vi "solar_voy_def Import (Item_Def).vi"(10 "Arguments":string[](array[string]), 11 "Item Tag":string) -> (1 "Valid?":bool, 2 "ID":u16, 3 "ITEM":T1)   [LabVIEW 2018]
doc: "This imports COSMOS parameter/item tag. Refer to: http://cosmosrb.com/docs/cmdtlm/\n\nSupported tags: \nPARAMETER\nARRAY_PARAMETER\nITEM, ARRAY_ITEM\nID_PARAMETER\nID_ITEM\nAPPEND_PARAMETER\nAPPEND_ARRAY_PARAMETER\nAPPEND_ARRAY_ITEM\nAPPEND_ID_PARAMETER\nAPPEND_ID_ITEM"
uses:
  type/solar_type Item Type.ctl
  solar_voy_def_ctl ITEM TYPE.ctl
  solar_voy_def_ctl ITEM.ctl
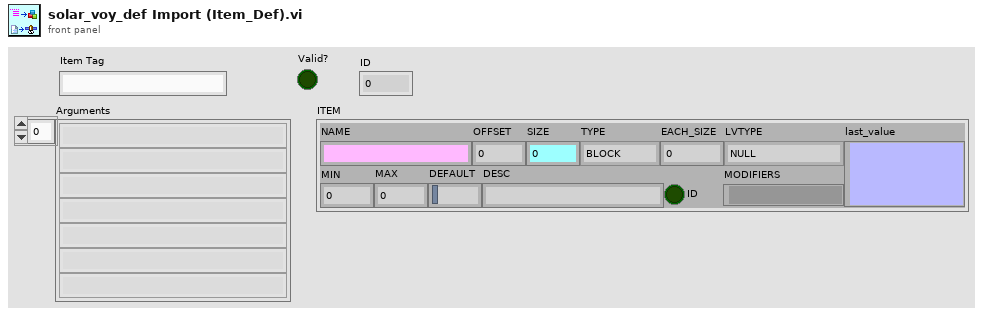
[diagram p1: front panel]
types:
  T1 = typedef "solar_voy_def_ctl ITEM.ctl" = cluster{"NAME":string, "OFFSET":i32, "SIZE":i32, "TYPE":T2, "EACH_SIZE":i32, "LVTYPE":T3, "MIN":dbl, "MAX":dbl, "DEFAULT":string, "DESC":string, "ID":bool, "MODIFIERS":variant, "last_value":variant}
  T2 = typedef "solar_voy_def_ctl ITEM TYPE.ctl" = enum8{"BLOCK", "INT", "UINT", "FLOAT", "STRING"}
  T3 = typedef "solar_type Item Type.ctl" = enum16{"NULL", "UNKNOWN", "CLUSTER", "I8", "I16", "I32", "I64", "U8", "U16", "U32", "U64", "U8_ENUM", "U16_ENUM", "U32_ENUM", "SGL", "DBL", "BOOLEAN", "STRING", "PATH", "VISA", "TAG", "TIME", "I8_1D", "I16_1D", "I32_1D", "I64_1D", "U8_1D", "U16_1D", "U32_1D", "U64_1D", "U8_ENUM_1D", "U16_ENUM_1D", "U32_ENUM_1D", "SGL_1D", "DBL_1D", "BOOLEAN_1D", "STRING_1D", "PATH_1D", "VISA_1D", "TAG_1D", "TIME_1D", "I8_2D", "I16_2D", "I32_2D", "I64_2D", "U8_2D", "U16_2D", "U32_2D", "U64_2D", "U8_ENUM_2D", "U16_ENUM_2D", "U32_ENUM_2D", "SGL_2D", "DBL_2D", "BOOLEAN_2D", "STRING_2D", "PATH_2D", "VISA_2D", "TAG_2D", "TIME_2D"}
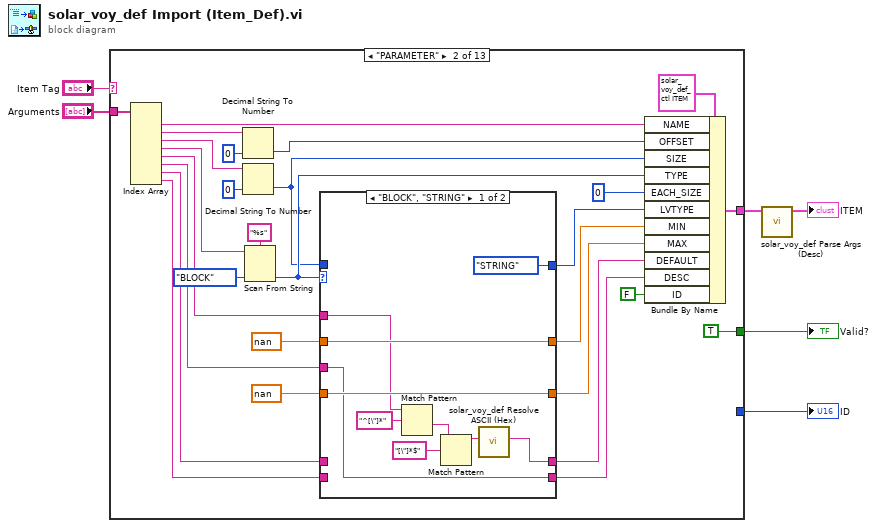
[diagram p0: block diagram]
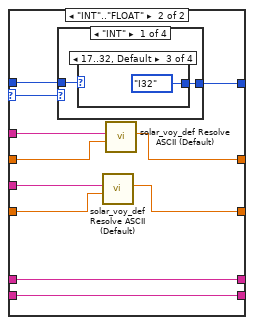
[diagram p3: hidden frame]
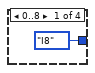
[diagram p4: hidden frame]
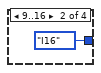
[diagram p5: hidden frame]
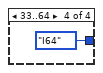
[diagram p6: hidden frame]
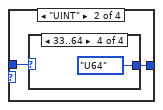
[diagram p7: hidden frame]
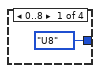
[diagram p8: hidden frame]
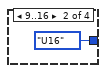
[diagram p9: hidden frame]
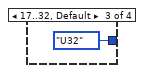
[diagram p10: hidden frame]
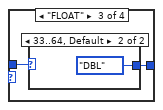
[diagram p11: hidden frame]
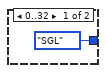
[diagram p12: hidden frame]
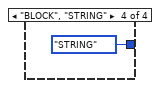
[diagram p13: hidden frame]
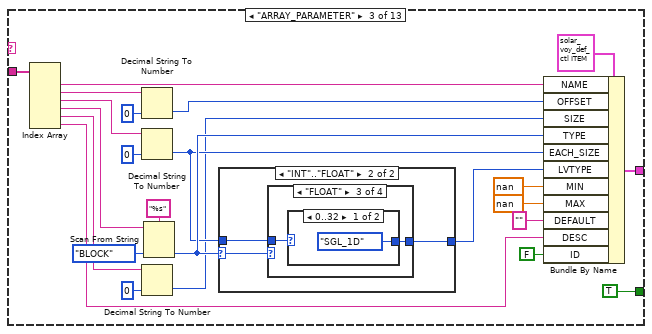
[diagram p14: hidden frame]
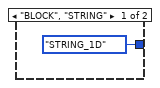
[diagram p15: hidden frame]
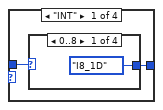
[diagram p16: hidden frame]
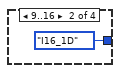
[diagram p17: hidden frame]
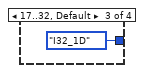
[diagram p18: hidden frame]
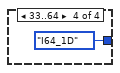
[diagram p19: hidden frame]
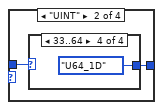
[diagram p20: hidden frame]
diagram:
  n1 = case shown="\"PARAMETER\"" "Item Tag" {
    tunnel: "Arguments" -> [_ w25 w93 w136 w181 w227 w299 w352 w418 w461 w502 w546 w616]
    tunnel: [_ w10 w84 w125 w172 w213 w288 w340 w412 w455 w494 w534 w608] -> w1
    tunnel: [_ TRUE TRUE TRUE TRUE TRUE TRUE TRUE TRUE TRUE TRUE TRUE TRUE] -> w4
    tunnel: [_ _ _ _ _ w206 w280 _ _ _ _ w526 w599] -> w3
    frame Default {
    }
    frame "PARAMETER" {
      n2 = Index Array(array=w25) -> (element #1=w24:string, element #2=w26:string, element #3=w27:string, element #4=w28:string, element #5=w29:string, element #6=w30:string, element #7=w32:string, element #8=w34:string)  [unwired: 8 in]
      n3 = Decimal String To Number(string=w26, default (0L)=0 ("OFFSET")) -> (number=w13:i32)  [unwired: 1 in, 1 out]
      n4 = Decimal String To Number(string=w27, default (0L)=0 ("OFFSET")) -> (number=w17:i32)  [unwired: 1 in, 1 out]
      n5 = Scan From String(format string="%s", input string=w28, default 1=solar_voy_def_ctl_ITEM_TYPE."BLOCK" ("TYPE")) -> (output 1=w22:T2)  [unwired: 2 in, 3 out]
      n6 = case shown="\"BLOCK\", \"STRING\"" w22 {
        selector: w22 -> [_ w53]
        tunnel: w17 -> [_ w55]
        tunnel: [solar_type_Item_Type."STRING" ("LVTYPE") w54] -> w18
        tunnel: nan ("MIN") -> [w43 w49]
        tunnel: [w43 w48] -> w20
        tunnel: nan ("MIN") -> [w42 w46]
        tunnel: [w42 w45] -> w23
        tunnel: w29 -> [w40 w50]
        tunnel: w30 -> [w41 w47]
        tunnel: [w35 w52] -> w31
        tunnel: w32 -> [_ w52]
        tunnel: [w41 w51] -> w33
        tunnel: w34 -> [_ w51]
        frame "BLOCK", "STRING" {
          n7 = Match Pattern(string=w40, regular expression="^[\"]*") -> (after substring=w38:string)  [unwired: 1 in, 3 out]
          n8 = Match Pattern(string=w38, regular expression="[\"]*$") -> (before substring=w36:string)  [unwired: 1 in, 3 out]
          n9 = call "solar_voy_def Resolve ASCII (Hex).vi"("DEFAULT (ASCII '\\xFF')"=w36) -> ("Resolved DEFAULT (Hex 'xFF')"=w35:string)  [unwired: 10 in]
        }
        frame "INT".."FLOAT" {
          n10 = case shown="\"INT\"" w53 {
            tunnel: w55 -> [w57 w63 w69 _]
            tunnel: [w56 w62 w68 solar_type_Item_Type."STRING" ("LVTYPE")] -> w54
            frame "INT" {
              n11 = case shown="17..32, Default" w57 {
                tunnel: [solar_type_Item_Type."I8" ("LVTYPE") solar_type_Item_Type."I16" ("LVTYPE") solar_type_Item_Type."I32" ("LVTYPE") solar_type_Item_Type."I64" ("LVTYPE")] -> w56
                frame 0..8 {
                }
                frame 9..16 {
                }
                frame 17..32, Default {
                }
                frame 33..64 {
                }
              }
            }
            frame "UINT" {
              n12 = case shown="33..64" w63 {
                tunnel: [solar_type_Item_Type."U8" ("LVTYPE") solar_type_Item_Type."U16" ("LVTYPE") solar_type_Item_Type."U32" ("LVTYPE") solar_type_Item_Type."U64" ("LVTYPE")] -> w62
                frame 0..8 {
                }
                frame 9..16 {
                }
                frame 17..32, Default {
                }
                frame 33..64 {
                }
              }
            }
            frame "FLOAT" {
              n13 = case shown="33..64, Default" w69 {
                tunnel: [solar_type_Item_Type."SGL" ("LVTYPE") solar_type_Item_Type."DBL" ("LVTYPE")] -> w68
                frame 0..32 {
                }
                frame 33..64, Default {
                }
              }
            }
            frame "BLOCK", "STRING" {
            }
          }
          n14 = call "solar_voy_def Resolve ASCII (Default).vi"("Default (NaN=Use Default)"=w46, "DEFAULT,MIN,MAX"=w47) -> ("DEFAULT,MIN,MAX out"=w45:dbl)  [unwired: 9 in]
          n15 = call "solar_voy_def Resolve ASCII (Default).vi"("Default (NaN=Use Default)"=w49, "DEFAULT,MIN,MAX"=w50) -> ("DEFAULT,MIN,MAX out"=w48:dbl)  [unwired: 9 in]
        }
      }
      n16 = Bundle By Name(cluster=T1 {"NAME"="", "OFFSET"=0, "SIZE"=0, "TYPE"=enum."BLOCK", "EACH_SIZE"=0, "LVTYPE"=enum."NULL", "MIN"=0.0, "MAX"=0.0, "DEFAULT"="", "DESC"="", "ID"=FALSE, "MODIFIERS"=variant, "last_value"=variant} ("element"), "NAME"=w24, "OFFSET"=w13, "SIZE"=w17, "TYPE"=w22, "EACH_SIZE"=0, "LVTYPE"=w18, "MIN"=w20, "MAX"=w23, "DEFAULT"=w31, "DESC"=w33, "ID"=FALSE) -> (w10:T1)
    }
    frame "ARRAY_PARAMETER" {
      n17 = Index Array(array=w93) -> (element #1=w92:string, element #2=w94:string, element #3=w95:string, element #4=w96:string, element #5=w78:string, element #6=w76:string)  [unwired: 6 in]
      n18 = Decimal String To Number(string=w94, default (0L)=0 ("OFFSET")) -> (number=w86:i32)  [unwired: 1 in, 1 out]
      n19 = Decimal String To Number(string=w95, default (0L)=0 ("OFFSET")) -> (number=w80:i32)  [unwired: 1 in, 1 out]
      n20 = Decimal String To Number(string=w78, default (0L)=0 ("OFFSET")) -> (number=w77:i32)  [unwired: 1 in, 1 out]
      n21 = Scan From String(format string="%s", input string=w96, default 1=solar_voy_def_ctl_ITEM_TYPE."BLOCK" ("TYPE")) -> (output 1=w91:T2)  [unwired: 2 in, 3 out]
      n22 = case shown="\"INT\"..\"FLOAT\"" w91 {
        selector: w91 -> [_ w98]
        tunnel: w80 -> [_ w100]
        tunnel: [solar_type_Item_Type."STRING_1D" ("LVTYPE") w99] -> w90
        frame "BLOCK", "STRING" {
        }
        frame "INT".."FLOAT" {
          n23 = case shown="\"FLOAT\"" w98 {
            tunnel: w100 -> [w102 w108 w114 _]
            tunnel: [w101 w107 w113 solar_type_Item_Type."STRING" ("LVTYPE")] -> w99
            frame "INT" {
              n24 = case shown="0..8" w102 {
                tunnel: [solar_type_Item_Type."I8_1D" ("LVTYPE") solar_type_Item_Type."I16_1D" ("LVTYPE") solar_type_Item_Type."I32_1D" ("LVTYPE") solar_type_Item_Type."I64_1D" ("LVTYPE")] -> w101
                frame 0..8 {
                }
                frame 9..16 {
                }
                frame 17..32, Default {
                }
                frame 33..64 {
                }
              }
            }
            frame "UINT" {
              n25 = case shown="33..64" w108 {
                tunnel: [solar_type_Item_Type."U8_1D" ("LVTYPE") solar_type_Item_Type."U16_1D" ("LVTYPE") solar_type_Item_Type."U32_1D" ("LVTYPE") solar_type_Item_Type."U64_1D" ("LVTYPE")] -> w107
                frame 0..8 {
                }
                frame 9..16 {
                }
                frame 17..32, Default {
                }
                frame 33..64 {
                }
              }
            }
            frame "FLOAT" {
              n26 = case shown="0..32" w114 {
                tunnel: [solar_type_Item_Type."SGL_1D" ("LVTYPE") solar_type_Item_Type."DBL_1D" ("LVTYPE")] -> w113
                frame 0..32 {
                }
                frame 33..64, Default {
                }
              }
            }
            frame "BLOCK", "STRING" {
            }
          }
        }
      }
      n27 = Bundle By Name(cluster=T1 {"NAME"="", "OFFSET"=0, "SIZE"=0, "TYPE"=enum."BLOCK", "EACH_SIZE"=0, "LVTYPE"=enum."NULL", "MIN"=0.0, "MAX"=0.0, "DEFAULT"="", "DESC"="", "ID"=FALSE, "MODIFIERS"=variant, "last_value"=variant} ("element"), "NAME"=w92, "OFFSET"=w86, "SIZE"=w77, "TYPE"=w91, "EACH_SIZE"=w80, "LVTYPE"=w90, "MIN"=nan, "MAX"=nan ("MIN"), "DEFAULT"="", "DESC"=w76, "ID"=FALSE) -> (w84:T1)
    }
    frame "ITEM" {
      n28 = Index Array(array=w136) -> (element #1=w135:string, element #2=w137:string, element #3=w138:string, element #4=w139:string, element #5=w118:string)  [unwired: 5 in]
      n29 = Decimal String To Number(string=w137, default (0L)=0 ("OFFSET")) -> (number=w128:i32)  [unwired: 1 in, 1 out]
      n30 = Decimal String To Number(string=w138, default (0L)=0 ("OFFSET")) -> (number=w132:i32)  [unwired: 1 in, 1 out]
      n31 = Scan From String(format string="%s", input string=w139, default 1=solar_voy_def_ctl_ITEM_TYPE."BLOCK" ("TYPE")) -> (output 1=w134:T2)  [unwired: 2 in, 3 out]
      n32 = case shown="\"INT\"..\"FLOAT\"" w134 {
        selector: w134 -> [_ w141]
        tunnel: w132 -> [_ w143]
        tunnel: [solar_type_Item_Type."STRING" ("LVTYPE") w142] -> w133
        frame "BLOCK", "STRING" {
        }
        frame "INT".."FLOAT" {
          n33 = case shown="\"INT\"" w141 {
            tunnel: w143 -> [w145 w151 w157 _]
            tunnel: [w144 w150 w156 solar_type_Item_Type."STRING" ("LVTYPE")] -> w142
            frame "INT" {
              n34 = case shown="17..32, Default" w145 {
                tunnel: [solar_type_Item_Type."I8" ("LVTYPE") solar_type_Item_Type."I16" ("LVTYPE") solar_type_Item_Type."I32" ("LVTYPE") solar_type_Item_Type."I64" ("LVTYPE")] -> w144
                frame 0..8 {
                }
                frame 9..16 {
                }
                frame 17..32, Default {
                }
                frame 33..64 {
                }
              }
            }
            frame "UINT" {
              n35 = case shown="33..64" w151 {
                tunnel: [solar_type_Item_Type."U8" ("LVTYPE") solar_type_Item_Type."U16" ("LVTYPE") solar_type_Item_Type."U32" ("LVTYPE") solar_type_Item_Type."U64" ("LVTYPE")] -> w150
                frame 0..8 {
                }
                frame 9..16 {
                }
                frame 17..32, Default {
                }
                frame 33..64 {
                }
              }
            }
            frame "FLOAT" {
              n36 = case shown="33..64, Default" w157 {
                tunnel: [solar_type_Item_Type."SGL" ("LVTYPE") solar_type_Item_Type."DBL" ("LVTYPE")] -> w156
                frame 0..32 {
                }
                frame 33..64, Default {
                }
              }
            }
            frame "BLOCK", "STRING" {
            }
          }
        }
      }
      n37 = Bundle By Name(cluster=T1 {"NAME"="", "OFFSET"=0, "SIZE"=0, "TYPE"=enum."BLOCK", "EACH_SIZE"=0, "LVTYPE"=enum."NULL", "MIN"=0.0, "MAX"=0.0, "DEFAULT"="", "DESC"="", "ID"=FALSE, "MODIFIERS"=variant, "last_value"=variant} ("element"), "NAME"=w135, "OFFSET"=w128, "SIZE"=w132, "TYPE"=w134, "EACH_SIZE"=0, "LVTYPE"=w133, "MIN"=nan, "MAX"=nan ("MIN"), "DEFAULT"="", "DESC"=w118, "ID"=FALSE) -> (w125:T1)
    }
    frame "ARRAY_ITEM" {
      n38 = Index Array(array=w181) -> (element #1=w180:string, element #2=w182:string, element #3=w183:string, element #4=w184:string, element #5=w166:string, element #6=w164:string)  [unwired: 6 in]
      n39 = Decimal String To Number(string=w182, default (0L)=0 ("OFFSET")) -> (number=w174:i32)  [unwired: 1 in, 1 out]
      n40 = Decimal String To Number(string=w183, default (0L)=0 ("OFFSET")) -> (number=w168:i32)  [unwired: 1 in, 1 out]
      n41 = Decimal String To Number(string=w166, default (0L)=0 ("OFFSET")) -> (number=w165:i32)  [unwired: 1 in, 1 out]
      n42 = Scan From String(format string="%s", input string=w184, default 1=solar_voy_def_ctl_ITEM_TYPE."BLOCK" ("TYPE")) -> (output 1=w179:T2)  [unwired: 2 in, 3 out]
      n43 = case shown="\"INT\"..\"FLOAT\"" w179 {
        selector: w179 -> [_ w186]
        tunnel: w168 -> [_ w188]
        tunnel: [solar_type_Item_Type."STRING_1D" ("LVTYPE") w187] -> w178
        frame "BLOCK", "STRING" {
        }
        frame "INT".."FLOAT" {
          n44 = case shown="\"FLOAT\"" w186 {
            tunnel: w188 -> [w190 w196 w202 _]
            tunnel: [w189 w195 w201 solar_type_Item_Type."STRING" ("LVTYPE")] -> w187
            frame "INT" {
              n45 = case shown="0..8" w190 {
                tunnel: [solar_type_Item_Type."I8_1D" ("LVTYPE") solar_type_Item_Type."I16_1D" ("LVTYPE") solar_type_Item_Type."I32_1D" ("LVTYPE") solar_type_Item_Type."I64_1D" ("LVTYPE")] -> w189
                frame 0..8 {
                }
                frame 9..16 {
                }
                frame 17..32, Default {
                }
                frame 33..64 {
                }
              }
            }
            frame "UINT" {
              n46 = case shown="33..64" w196 {
                tunnel: [solar_type_Item_Type."U8_1D" ("LVTYPE") solar_type_Item_Type."U16_1D" ("LVTYPE") solar_type_Item_Type."U32_1D" ("LVTYPE") solar_type_Item_Type."U64_1D" ("LVTYPE")] -> w195
                frame 0..8 {
                }
                frame 9..16 {
                }
                frame 17..32, Default {
                }
                frame 33..64 {
                }
              }
            }
            frame "FLOAT" {
              n47 = case shown="0..32" w202 {
                tunnel: [solar_type_Item_Type."SGL_1D" ("LVTYPE") solar_type_Item_Type."DBL_1D" ("LVTYPE")] -> w201
                frame 0..32 {
                }
                frame 33..64, Default {
                }
              }
            }
            frame "BLOCK", "STRING" {
            }
          }
        }
      }
      n48 = Bundle By Name(cluster=T1 {"NAME"="", "OFFSET"=0, "SIZE"=0, "TYPE"=enum."BLOCK", "EACH_SIZE"=0, "LVTYPE"=enum."NULL", "MIN"=0.0, "MAX"=0.0, "DEFAULT"="", "DESC"="", "ID"=FALSE, "MODIFIERS"=variant, "last_value"=variant} ("element"), "NAME"=w180, "OFFSET"=w174, "SIZE"=w165, "TYPE"=w179, "EACH_SIZE"=w168, "LVTYPE"=w178, "MIN"=nan, "MAX"=nan ("MIN"), "DEFAULT"="", "DESC"=w164, "ID"=FALSE) -> (w172:T1)
    }
    frame "ID_PARAMETER" {
      n49 = Index Array(array=w227) -> (element #1=w226:string, element #2=w228:string, element #3=w229:string, element #4=w230:string, element #5=w231:string, element #6=w232:string, element #7=w233:string, element #8=w235:string)  [unwired: 8 in]
      n50 = Decimal String To Number(string=w228, default (0L)=0 ("OFFSET")) -> (number=w216:i32)  [unwired: 1 in, 1 out]
      n51 = Decimal String To Number(string=w229, default (0L)=0 ("OFFSET")) -> (number=w209:i32)  [unwired: 1 in, 1 out]
      n52 = Scan From String(format string="%s", input string=w230, default 1=solar_voy_def_ctl_ITEM_TYPE."BLOCK" ("TYPE")) -> (output 1=w224:T2)  [unwired: 2 in, 3 out]
      n53 = case shown="\"BLOCK\", \"STRING\"" w224 {
        selector: w224 -> [_ w258]
        tunnel: w209 -> [_ w260]
        tunnel: [solar_type_Item_Type."STRING" ("LVTYPE") w259] -> w220
        tunnel: nan ("MIN") -> [w244 w255]
        tunnel: [w244 w254] -> w222
        tunnel: nan ("MIN") -> [w243 w252]
        tunnel: [w243 w251] -> w225
        tunnel: w231 -> [w238 w256]
        tunnel: w232 -> [w242 w253]
        tunnel: [w236 w246] -> w208
        tunnel: w233 -> [_ w247]
        tunnel: [w242 w257] -> w234
        tunnel: w235 -> [_ w257]
        frame "BLOCK", "STRING" {
          n54 = Match Pattern(string=w238, regular expression="^[\"]*") -> (after substring=w240:string)  [unwired: 1 in, 3 out]
          n55 = Match Pattern(string=w240, regular expression="[\"]*$") -> (before substring=w237:string)  [unwired: 1 in, 3 out]
          n56 = call "solar_voy_def Resolve ASCII (Hex).vi"("DEFAULT (ASCII '\\xFF')"=w237) -> ("Resolved DEFAULT (Hex 'xFF')"=w236:string)  [unwired: 10 in]
        }
        frame "INT".."FLOAT" {
          n57 = case shown="\"INT\"" w258 {
            tunnel: w260 -> [w262 w268 w274 _]
            tunnel: [w261 w267 w273 solar_type_Item_Type."STRING" ("LVTYPE")] -> w259
            frame "INT" {
              n58 = case shown="17..32, Default" w262 {
                tunnel: [solar_type_Item_Type."I8" ("LVTYPE") solar_type_Item_Type."I16" ("LVTYPE") solar_type_Item_Type."I32" ("LVTYPE") solar_type_Item_Type."I64" ("LVTYPE")] -> w261
                frame 0..8 {
                }
                frame 9..16 {
                }
                frame 17..32, Default {
                }
                frame 33..64 {
                }
              }
            }
            frame "UINT" {
              n59 = case shown="33..64" w268 {
                tunnel: [solar_type_Item_Type."U8" ("LVTYPE") solar_type_Item_Type."U16" ("LVTYPE") solar_type_Item_Type."U32" ("LVTYPE") solar_type_Item_Type."U64" ("LVTYPE")] -> w267
                frame 0..8 {
                }
                frame 9..16 {
                }
                frame 17..32, Default {
                }
                frame 33..64 {
                }
              }
            }
            frame "FLOAT" {
              n60 = case shown="33..64, Default" w274 {
                tunnel: [solar_type_Item_Type."SGL" ("LVTYPE") solar_type_Item_Type."DBL" ("LVTYPE")] -> w273
                frame 0..32 {
                }
                frame 33..64, Default {
                }
              }
            }
            frame "BLOCK", "STRING" {
            }
          }
          n61 = call "solar_voy_def Resolve ASCII (Default).vi"("Default (NaN=Use Default)"=w252, "DEFAULT,MIN,MAX"=w253) -> ("DEFAULT,MIN,MAX out"=w251:dbl)  [unwired: 9 in]
          n62 = call "solar_voy_def Resolve ASCII (Default).vi"("Default (NaN=Use Default)"=w255, "DEFAULT,MIN,MAX"=w256) -> ("DEFAULT,MIN,MAX out"=w254:dbl)  [unwired: 9 in]
          n63 = call "solar_voy_def Resolve ASCII (Default).vi"("Default (NaN=Use Default)"=0.0, "DEFAULT,MIN,MAX"=w247) -> ("DEFAULT,MIN,MAX out"=w249:dbl)  [unwired: 9 in]
          n64 = Format Into String(format string="%#f", w249) -> (resulting string=w246:string)  [unwired: 2 in, 1 out]
        }
      }
      n65 = Decimal String To Number(string=w208, default (0L)=u16 0 ("ID")) -> (number=w206:u16)  [unwired: 1 in, 1 out]
      n66 = Bundle By Name(cluster=T1 {"NAME"="", "OFFSET"=0, "SIZE"=0, "TYPE"=enum."BLOCK", "EACH_SIZE"=0, "LVTYPE"=enum."NULL", "MIN"=0.0, "MAX"=0.0, "DEFAULT"="", "DESC"="", "ID"=FALSE, "MODIFIERS"=variant, "last_value"=variant} ("element"), "NAME"=w226, "OFFSET"=w216, "SIZE"=w209, "TYPE"=w224, "EACH_SIZE"=0, "LVTYPE"=w220, "MIN"=w222, "MAX"=w225, "DEFAULT"=w208, "DESC"=w234, "ID"=TRUE) -> (w213:T1)
    }
    frame "ID_ITEM" {
      n67 = Index Array(array=w299) -> (element #1=w298:string, element #2=w300:string, element #3=w301:string, element #4=w302:string, element #5=w279:string, element #6=w282:string)  [unwired: 6 in]
      n68 = Decimal String To Number(string=w300, default (0L)=0 ("OFFSET")) -> (number=w291:i32)  [unwired: 1 in, 1 out]
      n69 = Decimal String To Number(string=w301, default (0L)=0 ("OFFSET")) -> (number=w295:i32)  [unwired: 1 in, 1 out]
      n70 = Scan From String(format string="%s", input string=w302, default 1=solar_voy_def_ctl_ITEM_TYPE."BLOCK" ("TYPE")) -> (output 1=w297:T2)  [unwired: 2 in, 3 out]
      n71 = case shown="\"BLOCK\", \"STRING\"" w297 {
        selector: w297 -> [_ w315]
        tunnel: w295 -> [_ w317]
        tunnel: [solar_type_Item_Type."STRING" ("LVTYPE") w316] -> w296
        tunnel: w279 -> [w304 w314]
        tunnel: [w303 w310] -> w278
        frame "BLOCK", "STRING" {
          # "Remove default quotes"
          n72 = Match Pattern(string=w304, regular expression="^[\"]*") -> (after substring=w306:string)  [unwired: 1 in, 3 out]
          n73 = Match Pattern(string=w306, regular expression="[\"]*$") -> (before substring=w308:string)  [unwired: 1 in, 3 out]
          n74 = call "solar_voy_def Resolve ASCII (Hex).vi"("DEFAULT (ASCII '\\xFF')"=w308) -> ("Resolved DEFAULT (Hex 'xFF')"=w303:string)  [unwired: 10 in]
        }
        frame "INT".."FLOAT" {
          n75 = case shown="\"INT\"" w315 {
            tunnel: w317 -> [w319 w325 w331 _]
            tunnel: [w318 w324 w330 solar_type_Item_Type."STRING" ("LVTYPE")] -> w316
            frame "INT" {
              n76 = case shown="17..32, Default" w319 {
                tunnel: [solar_type_Item_Type."I8" ("LVTYPE") solar_type_Item_Type."I16" ("LVTYPE") solar_type_Item_Type."I32" ("LVTYPE") solar_type_Item_Type."I64" ("LVTYPE")] -> w318
                frame 0..8 {
                }
                frame 9..16 {
                }
                frame 17..32, Default {
                }
                frame 33..64 {
                }
              }
            }
            frame "UINT" {
              n77 = case shown="33..64" w325 {
                tunnel: [solar_type_Item_Type."U8" ("LVTYPE") solar_type_Item_Type."U16" ("LVTYPE") solar_type_Item_Type."U32" ("LVTYPE") solar_type_Item_Type."U64" ("LVTYPE")] -> w324
                frame 0..8 {
                }
                frame 9..16 {
                }
                frame 17..32, Default {
                }
                frame 33..64 {
                }
              }
            }
            frame "FLOAT" {
              n78 = case shown="33..64, Default" w331 {
                tunnel: [solar_type_Item_Type."SGL" ("LVTYPE") solar_type_Item_Type."DBL" ("LVTYPE")] -> w330
                frame 0..32 {
                }
                frame 33..64, Default {
                }
              }
            }
            frame "BLOCK", "STRING" {
            }
          }
          n79 = call "solar_voy_def Resolve ASCII (Default).vi"("Default (NaN=Use Default)"=0.0, "DEFAULT,MIN,MAX"=w314) -> ("DEFAULT,MIN,MAX out"=w312:dbl)  [unwired: 9 in]
          n80 = Format Into String(format string="%#f", w312) -> (resulting string=w310:string)  [unwired: 2 in, 1 out]
        }
      }
      n81 = Decimal String To Number(string=w278, default (0L)=u16 0 ("ID")) -> (number=w280:u16)  [unwired: 1 in, 1 out]
      n82 = Bundle By Name(cluster=T1 {"NAME"="", "OFFSET"=0, "SIZE"=0, "TYPE"=enum."BLOCK", "EACH_SIZE"=0, "LVTYPE"=enum."NULL", "MIN"=0.0, "MAX"=0.0, "DEFAULT"="", "DESC"="", "ID"=FALSE, "MODIFIERS"=variant, "last_value"=variant} ("element"), "NAME"=w298, "OFFSET"=w291, "SIZE"=w295, "TYPE"=w297, "EACH_SIZE"=0, "LVTYPE"=w296, "MIN"=nan, "MAX"=nan ("MIN"), "DEFAULT"=w278, "DESC"=w282, "ID"=TRUE) -> (w288:T1)
    }
    frame "APPEND_PARAMETER" {
      # "no offset"
      n83 = Index Array(array=w352) -> (element #1=w336:string, element #2=w353:string, element #3=w354:string, element #4=w355:string, element #5=w356:string, element #6=w358:string, element #7=w360:string)  [unwired: 7 in]
      n84 = Decimal String To Number(string=w353, default (0L)=0 ("OFFSET")) -> (number=w345:i32)  [unwired: 1 in, 1 out]
      n85 = Scan From String(format string="%s", input string=w354, default 1=solar_voy_def_ctl_ITEM_TYPE."BLOCK" ("TYPE")) -> (output 1=w350:T2)  [unwired: 2 in, 3 out]
      n86 = case shown="\"BLOCK\", \"STRING\"" w350 {
        selector: w350 -> [_ w376]
        tunnel: w345 -> [_ w381]
        tunnel: [solar_type_Item_Type."STRING" ("LVTYPE") w380] -> w346
        tunnel: nan ("MIN") -> [w369 w379]
        tunnel: [w369 w378] -> w348
        tunnel: nan ("MIN") -> [w368 w377]
        tunnel: [w368 w375] -> w351
        tunnel: w355 -> [w363 w374]
        tunnel: w356 -> [w367 w373]
        tunnel: [w361 w371] -> w357
        tunnel: w358 -> [_ w371]
        tunnel: [w367 w372] -> w359
        tunnel: w360 -> [_ w372]
        frame "BLOCK", "STRING" {
          n87 = Match Pattern(string=w363, regular expression="^[\"]*") -> (after substring=w365:string)  [unwired: 1 in, 3 out]
          n88 = Match Pattern(string=w365, regular expression="[\"]*$") -> (before substring=w362:string)  [unwired: 1 in, 3 out]
          n89 = call "solar_voy_def Resolve ASCII (Hex).vi"("DEFAULT (ASCII '\\xFF')"=w362) -> ("Resolved DEFAULT (Hex 'xFF')"=w361:string)  [unwired: 10 in]
        }
        frame "INT".."FLOAT" {
          n90 = case shown="\"INT\"" w376 {
            tunnel: w381 -> [w383 w389 w395 _]
            tunnel: [w382 w388 w394 solar_type_Item_Type."STRING" ("LVTYPE")] -> w380
            frame "INT" {
              n91 = case shown="17..32, Default" w383 {
                tunnel: [solar_type_Item_Type."I8" ("LVTYPE") solar_type_Item_Type."I16" ("LVTYPE") solar_type_Item_Type."I32" ("LVTYPE") solar_type_Item_Type."I64" ("LVTYPE")] -> w382
                frame 0..8 {
                }
                frame 9..16 {
                }
                frame 17..32, Default {
                }
                frame 33..64 {
                }
              }
            }
            frame "UINT" {
              n92 = case shown="33..64" w389 {
                tunnel: [solar_type_Item_Type."U8" ("LVTYPE") solar_type_Item_Type."U16" ("LVTYPE") solar_type_Item_Type."U32" ("LVTYPE") solar_type_Item_Type."U64" ("LVTYPE")] -> w388
                frame 0..8 {
                }
                frame 9..16 {
                }
                frame 17..32, Default {
                }
                frame 33..64 {
                }
              }
            }
            frame "FLOAT" {
              n93 = case shown="33..64, Default" w395 {
                tunnel: [solar_type_Item_Type."SGL" ("LVTYPE") solar_type_Item_Type."DBL" ("LVTYPE")] -> w394
                frame 0..32 {
                }
                frame 33..64, Default {
                }
              }
            }
            frame "BLOCK", "STRING" {
            }
          }
          n94 = call "solar_voy_def Resolve ASCII (Default).vi"("Default (NaN=Use Default)"=w377, "DEFAULT,MIN,MAX"=w373) -> ("DEFAULT,MIN,MAX out"=w375:dbl)  [unwired: 9 in]
          n95 = call "solar_voy_def Resolve ASCII (Default).vi"("Default (NaN=Use Default)"=w379, "DEFAULT,MIN,MAX"=w374) -> ("DEFAULT,MIN,MAX out"=w378:dbl)  [unwired: 9 in]
        }
      }
      n96 = Bundle By Name(cluster=T1 {"NAME"="", "OFFSET"=0, "SIZE"=0, "TYPE"=enum."BLOCK", "EACH_SIZE"=0, "LVTYPE"=enum."NULL", "MIN"=0.0, "MAX"=0.0, "DEFAULT"="", "DESC"="", "ID"=FALSE, "MODIFIERS"=variant, "last_value"=variant} ("element"), "NAME"=w336, "OFFSET"=-1, "SIZE"=w345, "TYPE"=w350, "EACH_SIZE"=0, "LVTYPE"=w346, "MIN"=w348, "MAX"=w351, "DEFAULT"=w357, "DESC"=w359, "ID"=FALSE) -> (w340:T1)
    }
    frame "APPEND_ARRAY_PARAMETER" {
      # "no offset"
      n97 = Index Array(array=w418) -> (element #1=w399:string, element #2=w419:string, element #3=w420:string, element #4=w406:string, element #5=w404:string)  [unwired: 5 in]
      n98 = Decimal String To Number(string=w419, default (0L)=0 ("OFFSET")) -> (number=w408:i32)  [unwired: 1 in, 1 out]
      n99 = Decimal String To Number(string=w406, default (0L)=0 ("OFFSET")) -> (number=w405:i32)  [unwired: 1 in, 1 out]
      n100 = Scan From String(format string="%s", input string=w420, default 1=solar_voy_def_ctl_ITEM_TYPE."BLOCK" ("TYPE")) -> (output 1=w417:T2)  [unwired: 2 in, 3 out]
      n101 = case shown="\"INT\"..\"FLOAT\"" w417 {
        selector: w417 -> [_ w422]
        tunnel: w408 -> [_ w424]
        tunnel: [solar_type_Item_Type."STRING_1D" ("LVTYPE") w423] -> w416
        frame "BLOCK", "STRING" {
        }
        frame "INT".."FLOAT" {
          n102 = case shown="\"FLOAT\"" w422 {
            tunnel: w424 -> [w426 w432 w438 _]
            tunnel: [w425 w431 w437 solar_type_Item_Type."STRING" ("LVTYPE")] -> w423
            frame "INT" {
              n103 = case shown="0..8" w426 {
                tunnel: [solar_type_Item_Type."I8_1D" ("LVTYPE") solar_type_Item_Type."I16_1D" ("LVTYPE") solar_type_Item_Type."I32_1D" ("LVTYPE") solar_type_Item_Type."I64_1D" ("LVTYPE")] -> w425
                frame 0..8 {
                }
                frame 9..16 {
                }
                frame 17..32, Default {
                }
                frame 33..64 {
                }
              }
            }
            frame "UINT" {
              n104 = case shown="33..64" w432 {
                tunnel: [solar_type_Item_Type."U8_1D" ("LVTYPE") solar_type_Item_Type."U16_1D" ("LVTYPE") solar_type_Item_Type."U32_1D" ("LVTYPE") solar_type_Item_Type."U64_1D" ("LVTYPE")] -> w431
                frame 0..8 {
                }
                frame 9..16 {
                }
                frame 17..32, Default {
                }
                frame 33..64 {
                }
              }
            }
            frame "FLOAT" {
              n105 = case shown="0..32" w438 {
                tunnel: [solar_type_Item_Type."SGL_1D" ("LVTYPE") solar_type_Item_Type."DBL_1D" ("LVTYPE")] -> w437
                frame 0..32 {
                }
                frame 33..64, Default {
                }
              }
            }
            frame "BLOCK", "STRING" {
            }
          }
        }
      }
      n106 = Bundle By Name(cluster=T1 {"NAME"="", "OFFSET"=0, "SIZE"=0, "TYPE"=enum."BLOCK", "EACH_SIZE"=0, "LVTYPE"=enum."NULL", "MIN"=0.0, "MAX"=0.0, "DEFAULT"="", "DESC"="", "ID"=FALSE, "MODIFIERS"=variant, "last_value"=variant} ("element"), "NAME"=w399, "OFFSET"=-1, "SIZE"=w405, "TYPE"=w417, "EACH_SIZE"=w408, "LVTYPE"=w416, "MIN"=nan, "MAX"=nan ("MIN"), "DEFAULT"="", "DESC"=w404, "ID"=FALSE) -> (w412:T1)
    }
    frame "APPEND_ARRAY_ITEM" {
      # "no offset"
      n107 = Index Array(array=w461) -> (element #1=w442:string, element #2=w462:string, element #3=w463:string, element #4=w449:string, element #5=w447:string)  [unwired: 5 in]
      n108 = Decimal String To Number(string=w462, default (0L)=0 ("OFFSET")) -> (number=w451:i32)  [unwired: 1 in, 1 out]
      n109 = Decimal String To Number(string=w449, default (0L)=0 ("OFFSET")) -> (number=w448:i32)  [unwired: 1 in, 1 out]
      n110 = Scan From String(format string="%s", input string=w463, default 1=solar_voy_def_ctl_ITEM_TYPE."BLOCK" ("TYPE")) -> (output 1=w460:T2)  [unwired: 2 in, 3 out]
      n111 = case shown="\"INT\"..\"FLOAT\"" w460 {
        selector: w460 -> [_ w465]
        tunnel: w451 -> [_ w467]
        tunnel: [solar_type_Item_Type."STRING_1D" ("LVTYPE") w466] -> w459
        frame "BLOCK", "STRING" {
        }
        frame "INT".."FLOAT" {
          n112 = case shown="\"FLOAT\"" w465 {
            tunnel: w467 -> [w469 w475 w481 _]
            tunnel: [w468 w474 w480 solar_type_Item_Type."STRING" ("LVTYPE")] -> w466
            frame "INT" {
              n113 = case shown="0..8" w469 {
                tunnel: [solar_type_Item_Type."I8_1D" ("LVTYPE") solar_type_Item_Type."I16_1D" ("LVTYPE") solar_type_Item_Type."I32_1D" ("LVTYPE") solar_type_Item_Type."I64_1D" ("LVTYPE")] -> w468
                frame 0..8 {
                }
                frame 9..16 {
                }
                frame 17..32, Default {
                }
                frame 33..64 {
                }
              }
            }
            frame "UINT" {
              n114 = case shown="33..64" w475 {
                tunnel: [solar_type_Item_Type."U8_1D" ("LVTYPE") solar_type_Item_Type."U16_1D" ("LVTYPE") solar_type_Item_Type."U32_1D" ("LVTYPE") solar_type_Item_Type."U64_1D" ("LVTYPE")] -> w474
                frame 0..8 {
                }
                frame 9..16 {
                }
                frame 17..32, Default {
                }
                frame 33..64 {
                }
              }
            }
            frame "FLOAT" {
              n115 = case shown="0..32" w481 {
                tunnel: [solar_type_Item_Type."SGL_1D" ("LVTYPE") solar_type_Item_Type."DBL_1D" ("LVTYPE")] -> w480
                frame 0..32 {
                }
                frame 33..64, Default {
                }
              }
            }
            frame "BLOCK", "STRING" {
            }
          }
        }
      }
      n116 = Bundle By Name(cluster=T1 {"NAME"="", "OFFSET"=0, "SIZE"=0, "TYPE"=enum."BLOCK", "EACH_SIZE"=0, "LVTYPE"=enum."NULL", "MIN"=0.0, "MAX"=0.0, "DEFAULT"="", "DESC"="", "ID"=FALSE, "MODIFIERS"=variant, "last_value"=variant} ("element"), "NAME"=w442, "OFFSET"=-1, "SIZE"=w448, "TYPE"=w460, "EACH_SIZE"=w451, "LVTYPE"=w459, "MIN"=nan, "MAX"=nan ("MIN"), "DEFAULT"="", "DESC"=w447, "ID"=FALSE) -> (w455:T1)
    }
    frame "APPEND_ITEM" {
      n117 = Index Array(array=w502) -> (element #1=w486:string, element #2=w503:string, element #3=w504:string, element #4=w487:string)  [unwired: 4 in]
      n118 = Decimal String To Number(string=w503, default (0L)=0 ("OFFSET")) -> (number=w499:i32)  [unwired: 1 in, 1 out]
      n119 = Scan From String(format string="%s", input string=w504, default 1=solar_voy_def_ctl_ITEM_TYPE."BLOCK" ("TYPE")) -> (output 1=w501:T2)  [unwired: 2 in, 3 out]
      n120 = case shown="\"INT\"..\"FLOAT\"" w501 {
        selector: w501 -> [_ w506]
        tunnel: w499 -> [_ w508]
        tunnel: [solar_type_Item_Type."STRING" ("LVTYPE") w507] -> w500
        frame "BLOCK", "STRING" {
        }
        frame "INT".."FLOAT" {
          n121 = case shown="\"INT\"" w506 {
            tunnel: w508 -> [w510 w516 w522 _]
            tunnel: [w509 w515 w521 solar_type_Item_Type."STRING" ("LVTYPE")] -> w507
            frame "INT" {
              n122 = case shown="17..32, Default" w510 {
                tunnel: [solar_type_Item_Type."I8" ("LVTYPE") solar_type_Item_Type."I16" ("LVTYPE") solar_type_Item_Type."I32" ("LVTYPE") solar_type_Item_Type."I64" ("LVTYPE")] -> w509
                frame 0..8 {
                }
                frame 9..16 {
                }
                frame 17..32, Default {
                }
                frame 33..64 {
                }
              }
            }
            frame "UINT" {
              n123 = case shown="33..64" w516 {
                tunnel: [solar_type_Item_Type."U8" ("LVTYPE") solar_type_Item_Type."U16" ("LVTYPE") solar_type_Item_Type."U32" ("LVTYPE") solar_type_Item_Type."U64" ("LVTYPE")] -> w515
                frame 0..8 {
                }
                frame 9..16 {
                }
                frame 17..32, Default {
                }
                frame 33..64 {
                }
              }
            }
            frame "FLOAT" {
              n124 = case shown="33..64, Default" w522 {
                tunnel: [solar_type_Item_Type."SGL" ("LVTYPE") solar_type_Item_Type."DBL" ("LVTYPE")] -> w521
                frame 0..32 {
                }
                frame 33..64, Default {
                }
              }
            }
            frame "BLOCK", "STRING" {
            }
          }
        }
      }
      n125 = Bundle By Name(cluster=T1 {"NAME"="", "OFFSET"=0, "SIZE"=0, "TYPE"=enum."BLOCK", "EACH_SIZE"=0, "LVTYPE"=enum."NULL", "MIN"=0.0, "MAX"=0.0, "DEFAULT"="", "DESC"="", "ID"=FALSE, "MODIFIERS"=variant, "last_value"=variant} ("element"), "NAME"=w486, "OFFSET"=-1, "SIZE"=w499, "TYPE"=w501, "EACH_SIZE"=0, "LVTYPE"=w500, "MIN"=nan, "MAX"=nan ("MIN"), "DEFAULT"="", "DESC"=w487, "ID"=FALSE) -> (w494:T1)
    }
    frame "APPEND_ID_PARAMETER" {
      # "no offset"
      n126 = Index Array(array=w546) -> (element #1=w530:string, element #2=w547:string, element #3=w548:string, element #4=w549:string, element #5=w550:string, element #6=w551:string, element #7=w553:string)  [unwired: 7 in]
      n127 = Decimal String To Number(string=w547, default (0L)=0 ("OFFSET")) -> (number=w539:i32)  [unwired: 1 in, 1 out]
      n128 = Scan From String(format string="%s", input string=w548, default 1=solar_voy_def_ctl_ITEM_TYPE."BLOCK" ("TYPE")) -> (output 1=w544:T2)  [unwired: 2 in, 3 out]
      n129 = case shown="\"INT\"..\"FLOAT\"" w544 {
        selector: w544 -> [_ w576]
        tunnel: w539 -> [_ w578]
        tunnel: [solar_type_Item_Type."STRING" ("LVTYPE") w577] -> w540
        tunnel: nan ("MIN") -> [w562 w573]
        tunnel: [w562 w572] -> w542
        tunnel: nan ("MIN") -> [w561 w570]
        tunnel: [w561 w569] -> w545
        tunnel: w549 -> [w556 w574]
        tunnel: w550 -> [w560 w571]
        tunnel: [w554 w564] -> w527
        tunnel: w551 -> [_ w565]
        tunnel: [w560 w575] -> w552
        tunnel: w553 -> [_ w575]
        frame "BLOCK", "STRING" {
          n130 = Match Pattern(string=w556, regular expression="^[\"]*") -> (after substring=w558:string)  [unwired: 1 in, 3 out]
          n131 = Match Pattern(string=w558, regular expression="[\"]*$") -> (before substring=w555:string)  [unwired: 1 in, 3 out]
          n132 = call "solar_voy_def Resolve ASCII (Hex).vi"("DEFAULT (ASCII '\\xFF')"=w555) -> ("Resolved DEFAULT (Hex 'xFF')"=w554:string)  [unwired: 10 in]
        }
        frame "INT".."FLOAT" {
          n133 = case shown="\"INT\"" w576 {
            tunnel: w578 -> [w580 w586 w592 _]
            tunnel: [w579 w585 w591 solar_type_Item_Type."STRING" ("LVTYPE")] -> w577
            frame "INT" {
              n134 = case shown="17..32, Default" w580 {
                tunnel: [solar_type_Item_Type."I8" ("LVTYPE") solar_type_Item_Type."I16" ("LVTYPE") solar_type_Item_Type."I32" ("LVTYPE") solar_type_Item_Type."I64" ("LVTYPE")] -> w579
                frame 0..8 {
                }
                frame 9..16 {
                }
                frame 17..32, Default {
                }
                frame 33..64 {
                }
              }
            }
            frame "UINT" {
              n135 = case shown="33..64" w586 {
                tunnel: [solar_type_Item_Type."U8" ("LVTYPE") solar_type_Item_Type."U16" ("LVTYPE") solar_type_Item_Type."U32" ("LVTYPE") solar_type_Item_Type."U64" ("LVTYPE")] -> w585
                frame 0..8 {
                }
                frame 9..16 {
                }
                frame 17..32, Default {
                }
                frame 33..64 {
                }
              }
            }
            frame "FLOAT" {
              n136 = case shown="33..64, Default" w592 {
                tunnel: [solar_type_Item_Type."SGL" ("LVTYPE") solar_type_Item_Type."DBL" ("LVTYPE")] -> w591
                frame 0..32 {
                }
                frame 33..64, Default {
                }
              }
            }
            frame "BLOCK", "STRING" {
            }
          }
          n137 = call "solar_voy_def Resolve ASCII (Default).vi"("Default (NaN=Use Default)"=w573, "DEFAULT,MIN,MAX"=w574) -> ("DEFAULT,MIN,MAX out"=w572:dbl)  [unwired: 9 in]
          n138 = call "solar_voy_def Resolve ASCII (Default).vi"("Default (NaN=Use Default)"=w570, "DEFAULT,MIN,MAX"=w571) -> ("DEFAULT,MIN,MAX out"=w569:dbl)  [unwired: 9 in]
          n139 = call "solar_voy_def Resolve ASCII (Default).vi"("Default (NaN=Use Default)"=0.0, "DEFAULT,MIN,MAX"=w565) -> ("DEFAULT,MIN,MAX out"=w567:dbl)  [unwired: 9 in]
          n140 = Format Into String(format string="%#f", w567) -> (resulting string=w564:string)  [unwired: 2 in, 1 out]
        }
      }
      n141 = Bundle By Name(cluster=T1 {"NAME"="", "OFFSET"=0, "SIZE"=0, "TYPE"=enum."BLOCK", "EACH_SIZE"=0, "LVTYPE"=enum."NULL", "MIN"=0.0, "MAX"=0.0, "DEFAULT"="", "DESC"="", "ID"=FALSE, "MODIFIERS"=variant, "last_value"=variant} ("element"), "NAME"=w530, "OFFSET"=-1, "SIZE"=w539, "TYPE"=w544, "EACH_SIZE"=0, "LVTYPE"=w540, "MIN"=w542, "MAX"=w545, "DEFAULT"=w527, "DESC"=w552, "ID"=TRUE) -> (w534:T1)
      n142 = Decimal String To Number(string=w527, default (0L)=u16 0 ("ID")) -> (number=w526:u16)  [unwired: 1 in, 1 out]
    }
    frame "APPEND_ID_ITEM" {
      n143 = Index Array(array=w616) -> (element #1=w602:string, element #2=w617:string, element #3=w618:string, element #4=w597:string, element #5=w598:string)  [unwired: 5 in]
      n144 = Decimal String To Number(string=w617, default (0L)=0 ("OFFSET")) -> (number=w613:i32)  [unwired: 1 in, 1 out]
      n145 = Scan From String(format string="%s", input string=w618, default 1=solar_voy_def_ctl_ITEM_TYPE."BLOCK" ("TYPE")) -> (output 1=w615:T2)  [unwired: 2 in, 3 out]
      n146 = case shown="\"INT\"..\"FLOAT\"" w615 {
        selector: w615 -> [_ w631]
        tunnel: w613 -> [_ w633]
        tunnel: [solar_type_Item_Type."STRING" ("LVTYPE") w632] -> w614
        tunnel: w597 -> [w620 w627]
        tunnel: [w619 w626] -> w596
        frame "BLOCK", "STRING" {
          # "remove default quotes"
          n147 = Match Pattern(string=w620, regular expression="^[\"]*") -> (after substring=w623:string)  [unwired: 1 in, 3 out]
          n148 = Match Pattern(string=w623, regular expression="[\"]*$") -> (before substring=w621:string)  [unwired: 1 in, 3 out]
          n149 = call "solar_voy_def Resolve ASCII (Hex).vi"("DEFAULT (ASCII '\\xFF')"=w621) -> ("Resolved DEFAULT (Hex 'xFF')"=w619:string)  [unwired: 10 in]
        }
        frame "INT".."FLOAT" {
          n150 = case shown="\"INT\"" w631 {
            tunnel: w633 -> [w635 w641 w647 _]
            tunnel: [w634 w640 w646 solar_type_Item_Type."STRING" ("LVTYPE")] -> w632
            frame "INT" {
              n151 = case shown="17..32, Default" w635 {
                tunnel: [solar_type_Item_Type."I8" ("LVTYPE") solar_type_Item_Type."I16" ("LVTYPE") solar_type_Item_Type."I32" ("LVTYPE") solar_type_Item_Type."I64" ("LVTYPE")] -> w634
                frame 0..8 {
                }
                frame 9..16 {
                }
                frame 17..32, Default {
                }
                frame 33..64 {
                }
              }
            }
            frame "UINT" {
              n152 = case shown="33..64" w641 {
                tunnel: [solar_type_Item_Type."U8" ("LVTYPE") solar_type_Item_Type."U16" ("LVTYPE") solar_type_Item_Type."U32" ("LVTYPE") solar_type_Item_Type."U64" ("LVTYPE")] -> w640
                frame 0..8 {
                }
                frame 9..16 {
                }
                frame 17..32, Default {
                }
                frame 33..64 {
                }
              }
            }
            frame "FLOAT" {
              n153 = case shown="33..64, Default" w647 {
                tunnel: [solar_type_Item_Type."SGL" ("LVTYPE") solar_type_Item_Type."DBL" ("LVTYPE")] -> w646
                frame 0..32 {
                }
                frame 33..64, Default {
                }
              }
            }
            frame "BLOCK", "STRING" {
            }
          }
          n154 = call "solar_voy_def Resolve ASCII (Default).vi"("Default (NaN=Use Default)"=0.0, "DEFAULT,MIN,MAX"=w627) -> ("DEFAULT,MIN,MAX out"=w629:dbl)  [unwired: 9 in]
          n155 = Format Into String(format string="%#f", w629) -> (resulting string=w626:string)  [unwired: 2 in, 1 out]
        }
      }
      n156 = Bundle By Name(cluster=T1 {"NAME"="", "OFFSET"=0, "SIZE"=0, "TYPE"=enum."BLOCK", "EACH_SIZE"=0, "LVTYPE"=enum."NULL", "MIN"=0.0, "MAX"=0.0, "DEFAULT"="", "DESC"="", "ID"=FALSE, "MODIFIERS"=variant, "last_value"=variant} ("element"), "NAME"=w602, "OFFSET"=-1, "SIZE"=w613, "TYPE"=w615, "EACH_SIZE"=0, "LVTYPE"=w614, "MIN"=nan, "MAX"=nan ("MIN"), "DEFAULT"=w596, "DESC"=w598, "ID"=TRUE) -> (w608:T1)
      n157 = Decimal String To Number(string=w596, default (0L)=u16 0 ("ID")) -> (number=w599:u16)  [unwired: 1 in, 1 out]
    }
  }
  "Valid?" <- w4
  "ID" <- w3
  n158 = call "solar_voy_def Parse Args (Desc).vi"("Default ITEM"=w1) -> ("ITEM out"=→"ITEM":T1)  [unwired: 10 in]
